vi "Lockin_AIWFM_time.vi"(8 "error in (no error)":errorcluster, 11 "Transport":refnum<class "SMO.Transport.lvclass">) -> (0 "error out":errorcluster, 3 "Transport out":refnum<class "SMO.Transport.lvclass">)   [LabVIEW 2019, in "SMO.Transport.lvclass"]
uses:
  SMO.Transport.lvclass
  <userlib>/LevyLab/Instrument Framework/Instrument Types/Cryostat/Instrument.Cryostat.lvclass
  SMO.Control Experiment/SMO.Control Experiment.lvclass
  <userlib>/LevyLab/Lockin-Multichannel/Instrument.Lockin/Instrument.Lockin.lvclass
  <userlib>/LevyLab/Krohn Hite 7008/Instrument.KH7008.lvclass
  SMO.Control Experiment/Private/Control Experiment SM/Typedefs/Instruments--cluster.ctl
  <userlib>/LevyLab/Instrument Framework/Instrument Types/VSource/Instrument.VSource.lvclass
  <userlib>/LevyLab/Instrument Framework/Instrument Types/VNA/Instrument.VNA.lvclass
  <userlib>/LevyLab/Instrument Framework/Instrument Types/Strain/Instrument.Strain.lvclass
  <userlib>/LevyLab/Instrument Framework/Instrument Types/CBridge/Instrument.CBridge.lvclass
  <vilib>/Waveform/WDTOps.llb/WDT Append Waveforms DBL.vi
  <userlib>/LevyLab/XY Utilities/xy_utilities.lvlib
  <userlib>/LevyLab/XY Utilities/subVIs/Waveform to XY (single).vi
  <userlib>/LevyLab/XY Utilities/subVIs/Get X and Y (single).vi
  <userlib>/LevyLab/Instrument Framework/Instrument Types/Delay Line/Instrument.DelayLine.lvclass
panel:
  in  "Stop":bool
  in  "Tab Control":enum32{"Control", "Waveform", "Other"}(tab)
  in  "wait (ms)":u32=1000
  in  "Experiment Description":string="cool down\n\n"
  in  "Experiment Folder":string="cooldown"
  out "AI":cluster{dbl[], dbl[]}[](graph)
  # "*** These controls are only read if this VI is the top level. If is is called from Sweep Control then the folder and comments come from Sweep Control.vi ***"
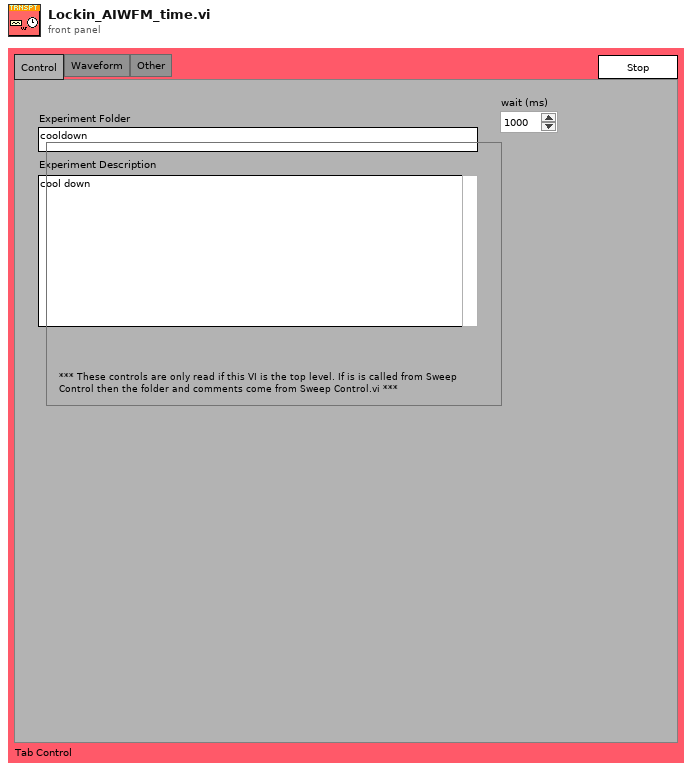
[diagram p1: front panel]
types:
  T1 = enum32{"Invalid", "Standard", "Closed", "Hidden", "Minimized", "Maximized"}
  T2 = enum32{"invalid app kind", "Development System", "Run Time System", "Student Edition", "Embedded LabVIEW", "Evaluation", "Custom"}
  T3 = typedef "SMO.Control Experiment.lvclass/Instruments--cluster.ctl" = cluster{"Lockin":refnum<class "Instrument.Lockin.lvclass">, "Temperature":refnum<class "Instrument.Cryostat.lvclass">, "Magnet":refnum<class "Instrument.Cryostat.lvclass">, "Rotator":refnum<class "Instrument.Cryostat.lvclass">, "Level":refnum<class "Instrument.Cryostat.lvclass">, "C Bridge":refnum<class "Instrument.CBridge.lvclass">, "Optical Delay Line":refnum<class "Instrument.DelayLine.lvclass">, "Strain Cell":refnum<class "Instrument.Strain.lvclass">, "VNA":refnum<class "Instrument.VNA.lvclass">, "Voltage Source":refnum<class "Instrument.VSource.lvclass">, "KH7008":refnum<class "Instrument.KH7008.lvclass">[]}
  T4 = cluster{"Core":cluster{"Current VI Reference":refnum<vi>, "Close Panel on Exit?":bool}, "Transport":refnum<class "SMO.Transport.lvclass">, "Control Experiment":refnum<class "SMO.Control Experiment.lvclass">, "Notifier":refnum<notifier>, "Instruments":T3, "path":path, "time":dbl, "temperature":dbl, "magnet field":dbl, "AI XY (new)":cluster{dbl[], dbl[]}[], "AI XY (all)":cluster{dbl[], dbl[]}[], "AI Waveform (s)":waveform(dbl)[], "t0":timestamp, "Execution:State":enum32{"Bad", "Idle", "Run top level", "Running"}}
  T5 = enum32{"Bad", "Idle", "Run top level", "Running"}
  T6 = cluster{"Current VI Reference":refnum<vi>, "Close Panel on Exit?":bool}
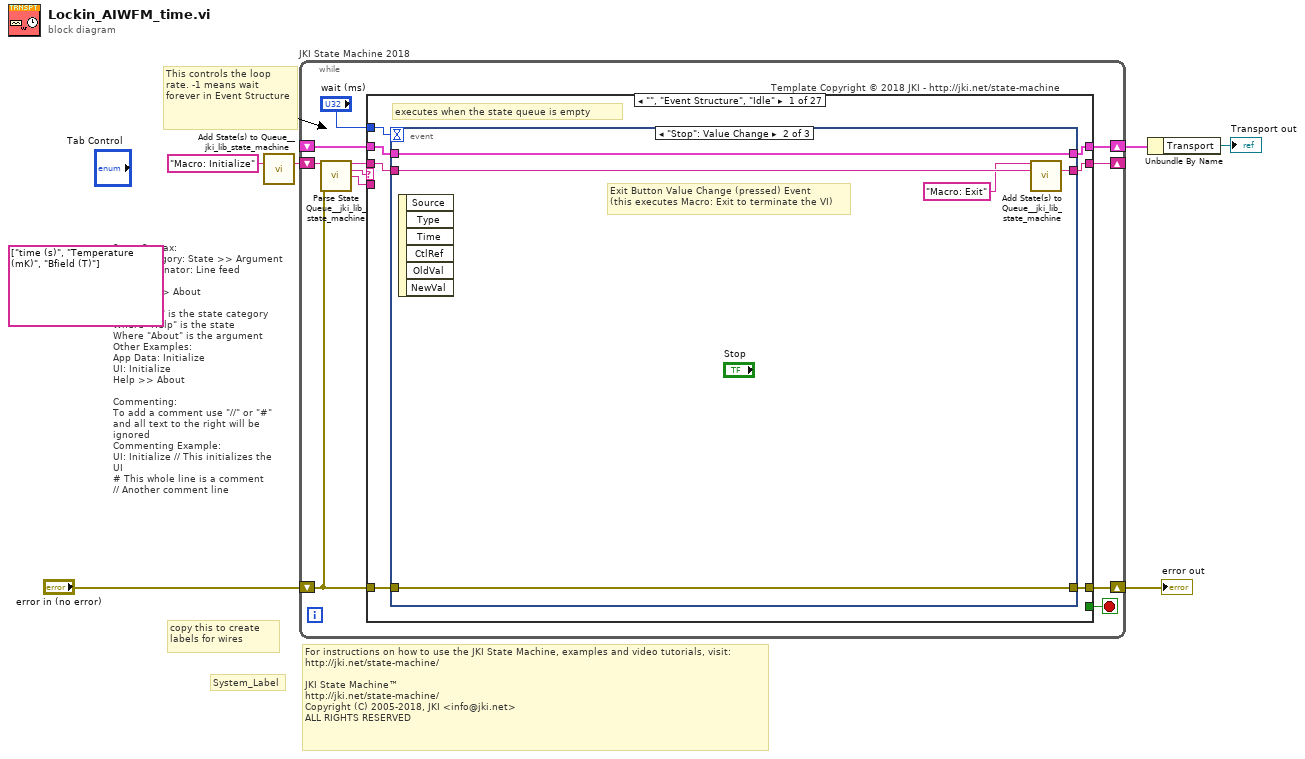
[diagram p0: block diagram]
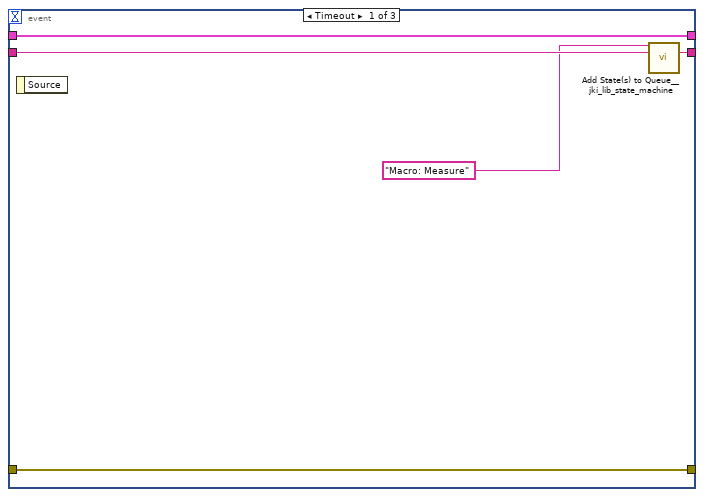
[diagram p2: hidden frame]
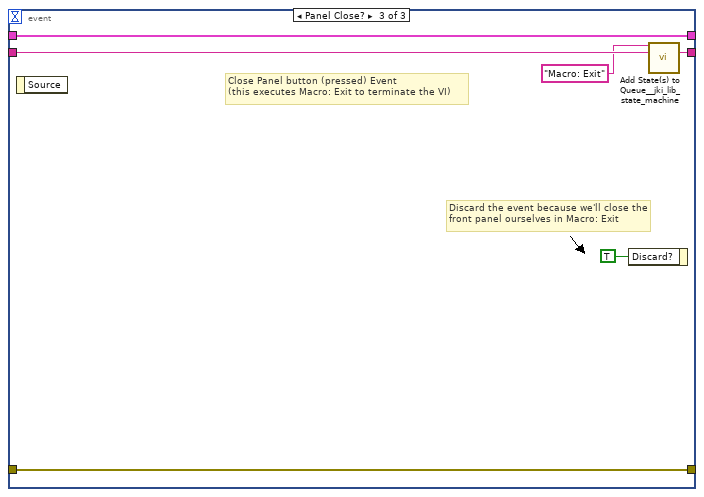
[diagram p3: hidden frame]
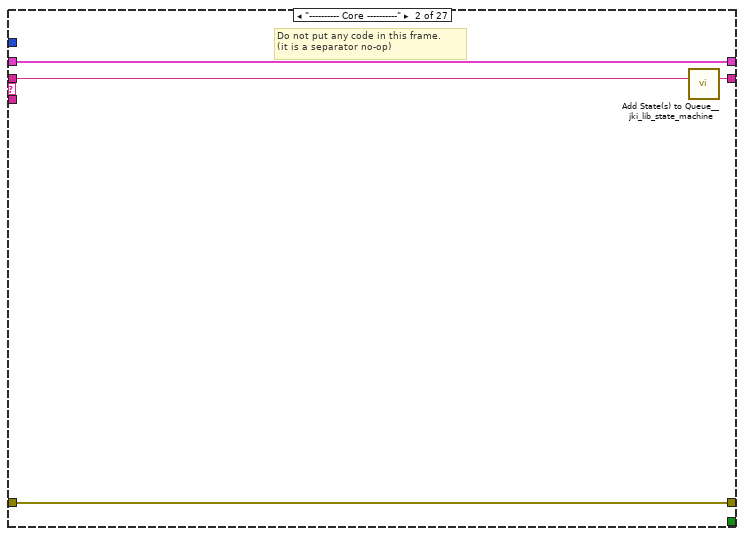
[diagram p4: hidden frame]
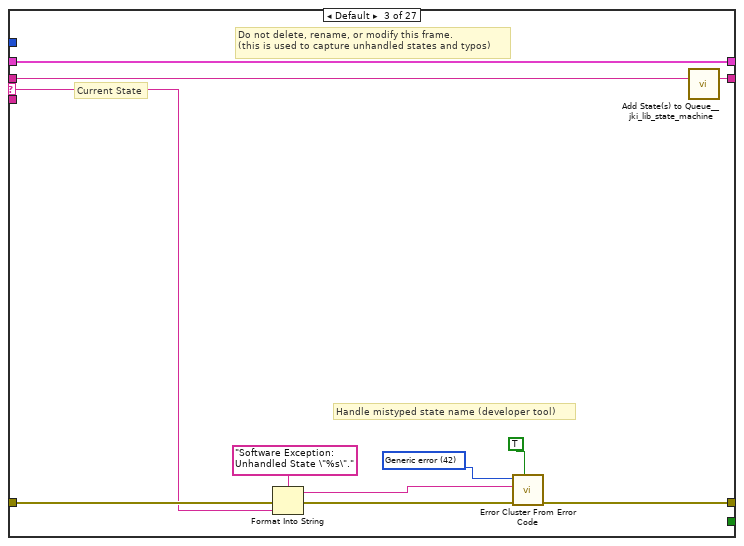
[diagram p5: hidden frame]
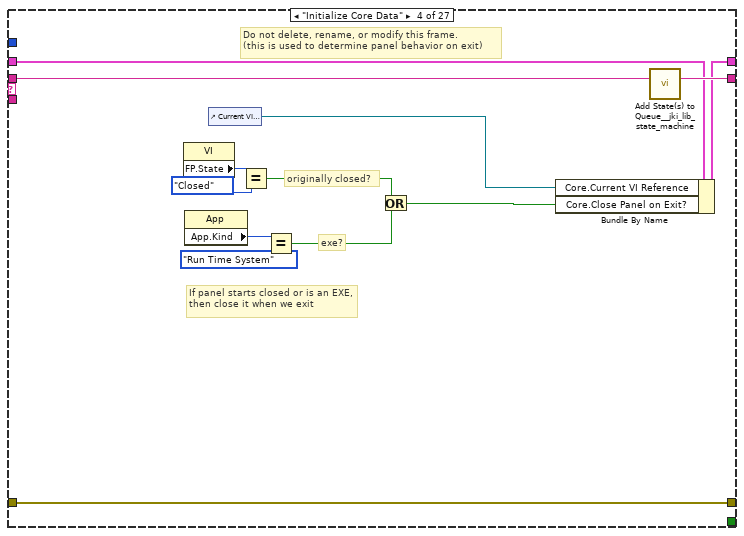
[diagram p6: hidden frame]
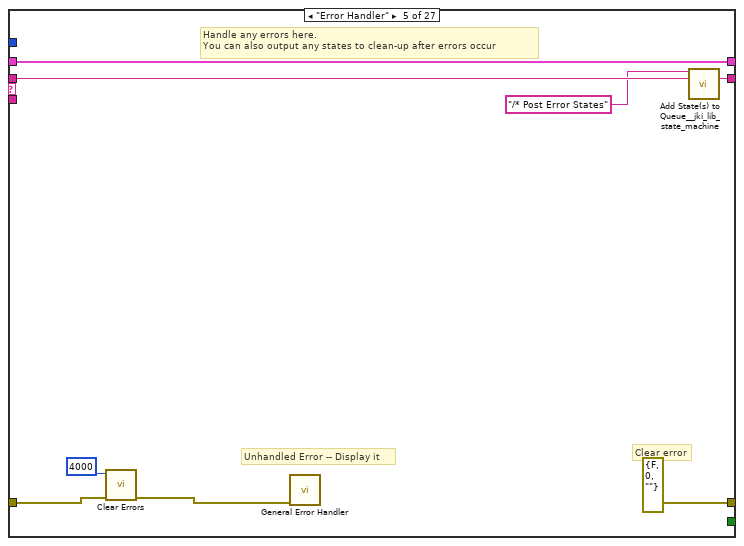
[diagram p7: hidden frame]
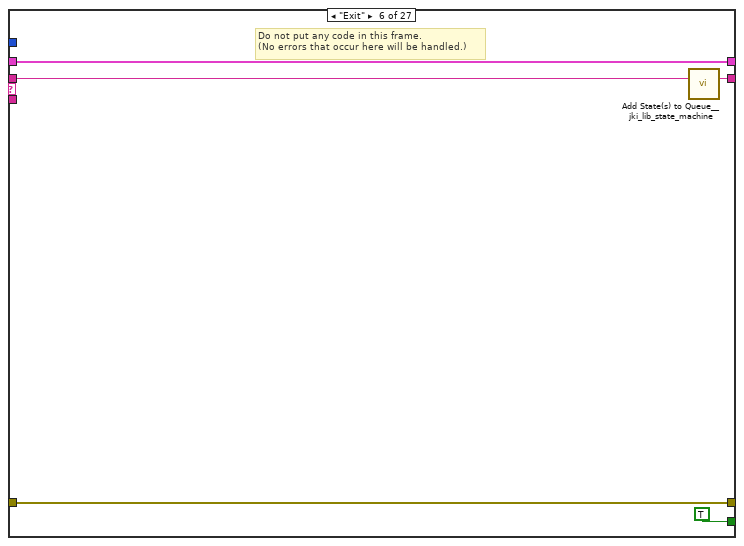
[diagram p8: hidden frame]
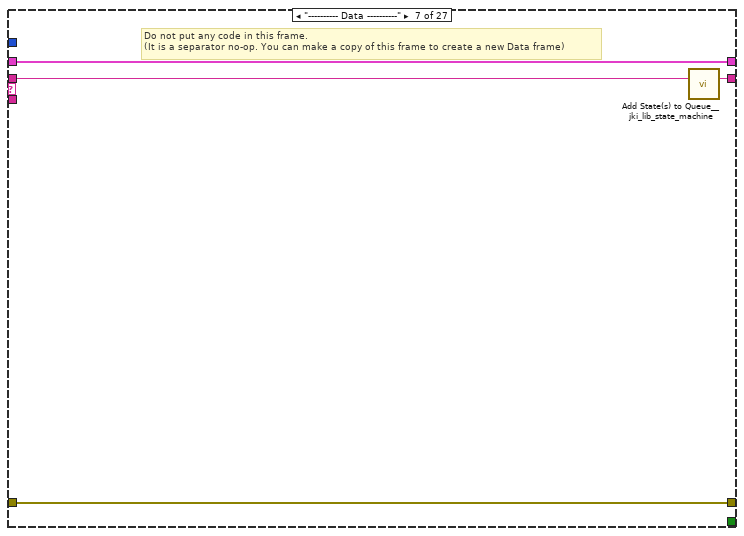
[diagram p9: hidden frame]
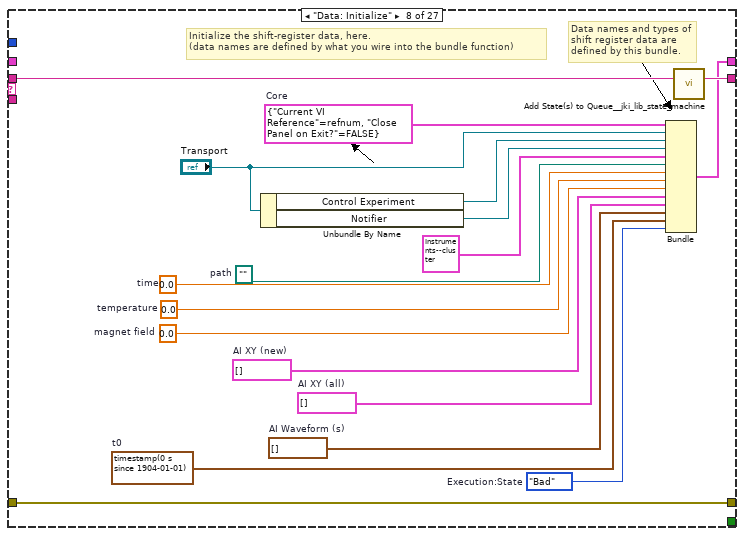
[diagram p10: hidden frame]
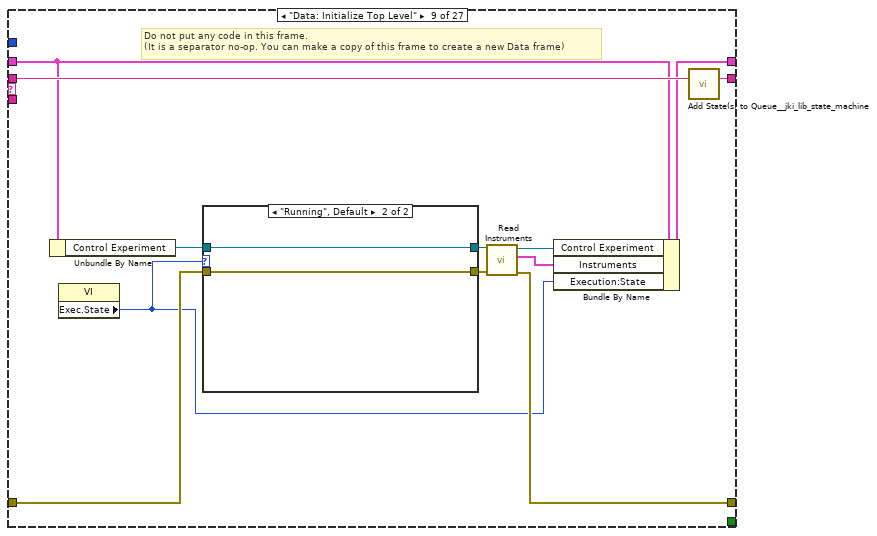
[diagram p11: hidden frame]
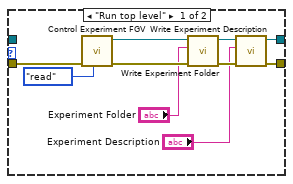
[diagram p12: hidden frame]
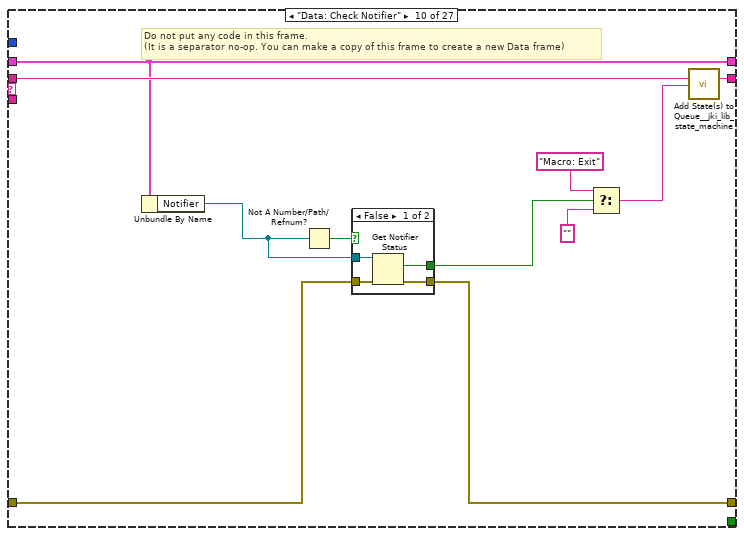
[diagram p13: hidden frame]
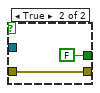
[diagram p14: hidden frame]
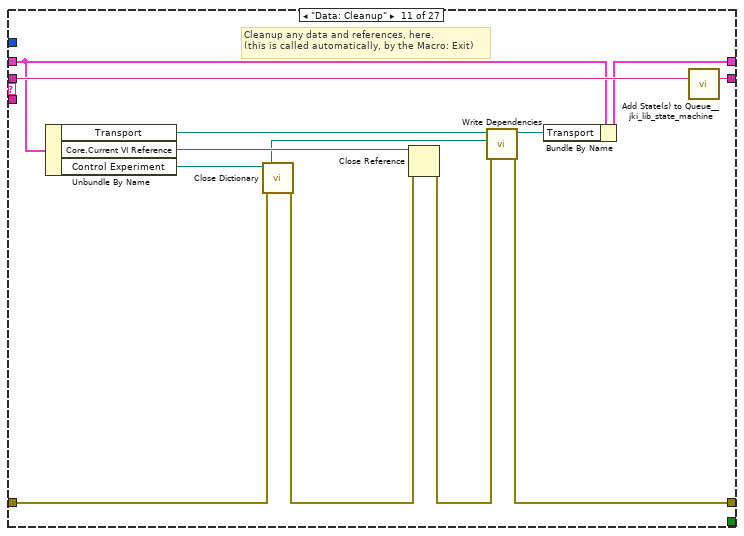
[diagram p15: hidden frame]
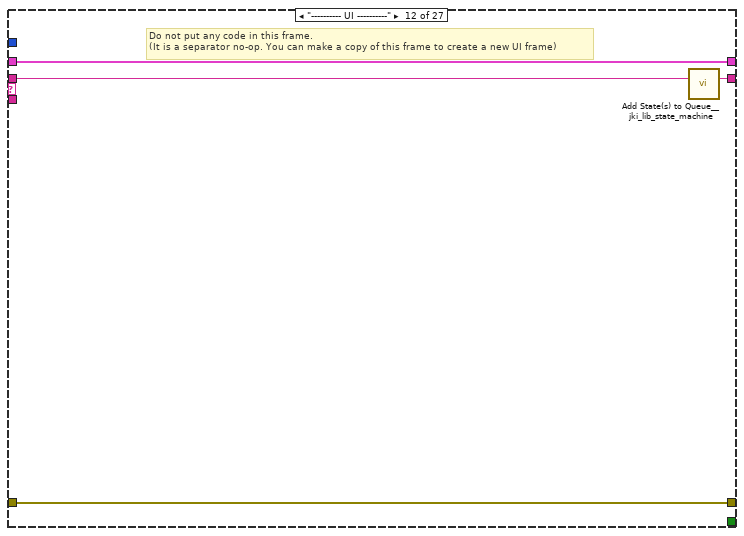
[diagram p16: hidden frame]
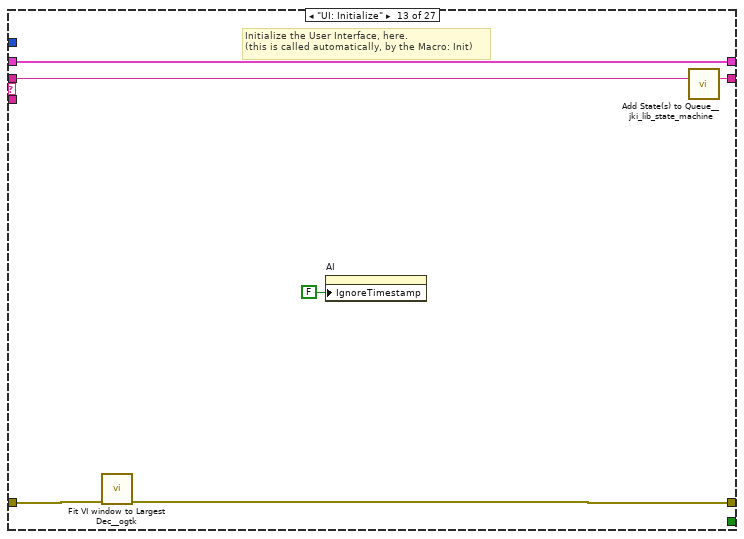
[diagram p17: hidden frame]
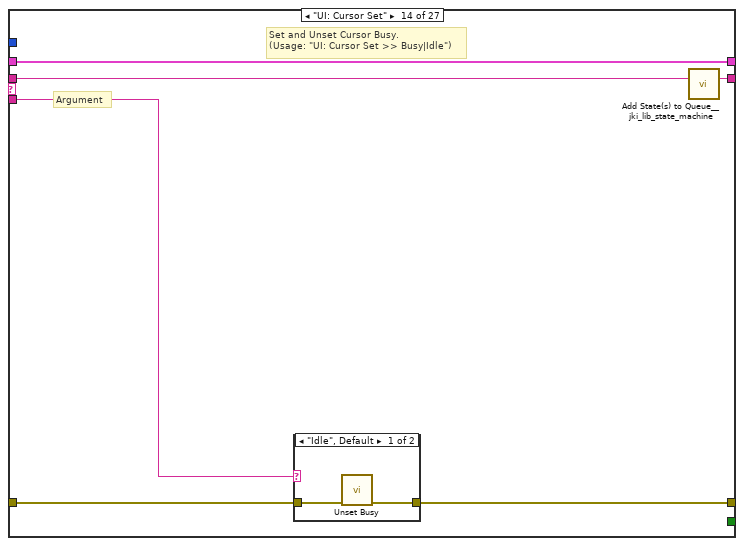
[diagram p18: hidden frame]
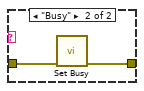
[diagram p19: hidden frame]
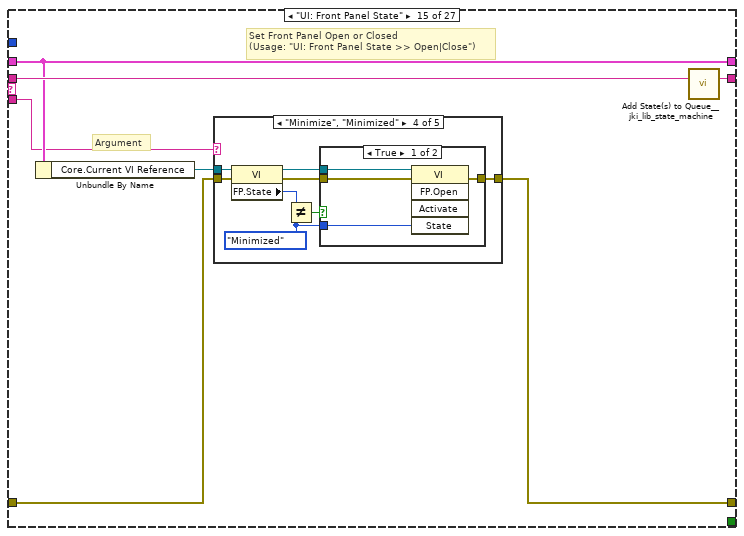
[diagram p20: hidden frame]
diagram:
  (unwired) string[] ["time (s)", "Temperature (mK)", "Bfield (T)"] ("wavenames (.Vx, etc)")
  # "For instructions on how to use the JKI State Machine, examples and video tutorials, visit:\nhttp://jki.net/state-machine/\n\nJKI State Machine™\nhttp://jki.net/state-machine/\nCopyright (C) 2005-2018, JKI <info@jki.net>\nALL RIGHTS RESERVED"
  # "State Syntax:\nStateCategory: State >> Argument\nLine Terminator: Line feed\nExample:\nUI: Help >> About\n\nWhere \"UI\" is the state category\nWhere \"Help\" is the state\nWhere \"About\" is the argument\nOther Examples:\nApp Data: Initialize\nUI: Initialize\nHelp >> About\n\nCommenting:\nTo add a comment use \"//\" or \"#\" and all text to the right will be ignored\nCommenting Example:\nUI: Initialize // This initializes the UI\n# This whole line is a comment\n// Another comment line"
  # "copy this to create labels for wires"
  # "This controls the loop rate. -1 means wait forever in Event Structure"
  # "System_Label"
  n1 = call <vilib>:"Add State(s) to Queue__jki_lib_state_machine.vi"("State(s) in (\"\")"="Macro: Initialize") -> ("States Out"=w6:string)  [unwired: 14 in]
  n2 = while "JKI State Machine 2018" {
    shift-right: [w10] -> w2
    shift-left: _ -> [w9]
    shift-right: [w13] -> w3
    shift-left: "error in (no error)" -> [w8]
    shift-right: [w12] -> _
    shift-left: w6 -> [w14]
    stop <- w11 stop-if-true
    # "Template Copyright © 2018 JKI - http://jki.net/state-machine"
    n3 = call <vilib>:"Parse State Queue__jki_lib_state_machine.vi"("State Queue"=w14, "Error In (no error)"=w8) -> ("Remaining States"=w16:string, "Current State"=w17:string, "Arguments"=w15:string)  [unwired: 11 in]
    n4 = case shown="\"\", \"Event Structure\", \"Idle\"" w17 {
      selector: w17 -> [_ _ w45 _ _ _ _ _ _ _ _ _ _ _ _ _ _ _ _ _ _ _ _ _ _ _ _]
      tunnel: w16 -> [w24 w44 w49 w68 w76 w81 w85 w103 w115 w138 w157 w161 w167 w173 w184 w254 w258 w263 w271 w281 w285 w299 w323 w334 w346 w358 w370]
      tunnel: w15 -> [_ _ _ _ _ _ _ _ _ _ _ _ _ w168 w178 _ _ _ _ _ _ _ _ _ _ _ _]
      tunnel: w9 -> [w22 w41 w47 w61 w73 w79 w82 _ w111 w135 w147 w158 w165 w171 w180 w252 w255 w260 w268 w278 w282 w287 w320 w330 w342 w356 w367]
      tunnel: [w21 w42 w51 w65 errorcluster {"status"=FALSE, "code"=0, "source"=""} ("error out") w78 w83 w100 w105 w133 w148 w159 w163 w169 w181 w251 w256 w261 w269 w279 w283 w297 w321 w324 w335 w351 w361] -> w13
      tunnel: w8 -> [w20 w42 w50 w65 w70 w78 w83 w100 w110 w132 w153 w159 w164 w170 w182 w251 w256 w261 w269 w279 w283 w292 w321 w327 w343 w350 w362]
      tunnel: [w23 w43 w48 w67 w75 w80 w84 w102 w114 w137 w156 w160 w166 w172 w183 w253 w257 w262 w270 w280 w284 w298 w322 w333 w345 w357 w369] -> w12
      tunnel: [_ _ _ _ _ TRUE _ _ _ _ _ _ _ _ _ _ _ _ _ _ _ _ _ _ _ _ _] -> w11
      tunnel: [w19 w41 w47 w66 w73 w79 w82 w101 w112 w135 w146 w158 w165 w171 w180 w252 w255 w260 w268 w278 w282 w286 w320 w331 w341 w355 w368] -> w10
      tunnel: "wait (ms)" -> [w18 _ _ _ _ _ _ _ _ _ _ _ _ _ _ _ _ _ _ _ _ _ _ _ _ _ _]
      frame "", "Event Structure", "Idle" {
        # "executes when the state queue is empty"
        n5 = event shown="[1] \"Stop\": Value Change" {
          selector: _ -> [_ _ _]
          dyn-events: _ -> [_ _ _]
          timeout: w18 -> [_ _ _]
          tunnel: w24 -> [w29 w34 w40]
          tunnel: [w28 w33 w39] -> w23
          tunnel: w22 -> [w26 w31 w37]
          tunnel: [w27 w32 w38] -> w21
          tunnel: w20 -> [w27 w32 w38]
          tunnel: [w26 w31 w37] -> w19
          event Timeout {
            n6 = event-data() -> ()  [unwired: 1 in, 1 out]
            n7 = call <vilib>:"Add State(s) to Queue__jki_lib_state_machine.vi"("State(s) in Front (\"\")"="Macro: Measure" ("State(s) in Front (\"\")"), "State(s) in (\"\")"=w29) -> ("States Out"=w28:string)  [unwired: 13 in]
          }
          event "Stop": Value Change {
            # "Exit Button Value Change (pressed) Event\n(this executes Macro: Exit to terminate the VI)"
            n8 = event-data() -> ()  [unwired: 1 in, 6 out]
            n9 = call <vilib>:"Add State(s) to Queue__jki_lib_state_machine.vi"("State(s) in Front (\"\")"="Macro: Exit", "State(s) in (\"\")"=w34) -> ("States Out"=w33:string)  [unwired: 13 in]
          }
          event Panel Close? {
            # "Discard the event because we'll close the front panel ourselves in Macro: Exit"
            # "Close Panel button (pressed) Event\n(this executes Macro: Exit to terminate the VI)"
            n10 = event-data() -> ()  [unwired: 1 in, 1 out]
            n11 = event-data("Discard?"=TRUE) -> ()  [unwired: 1 in, 1 out]
            n12 = call <vilib>:"Add State(s) to Queue__jki_lib_state_machine.vi"("State(s) in Front (\"\")"="Macro: Exit", "State(s) in (\"\")"=w40) -> ("States Out"=w39:string)  [unwired: 13 in]
          }
        }
      }
      frame "---------- Core ----------" {
        # "Do not put any code in this frame.\n(it is a separator no-op)"
        n13 = call <vilib>:"Add State(s) to Queue__jki_lib_state_machine.vi"("State(s) in (\"\")"=w44) -> ("States Out"=w43:string)  [unwired: 14 in]
      }
      frame Default {
        w54 = 42 items=["No error", "Argument error", "Memory is full", "Out of zone", "End of file", "File already open", "Generic file I/O error", "File not found", "File permission error", "Disk is full", "Duplicate path", "Too many files open", "System feature not enabled", "Resource file not found", "Cannot add resource", "Resource not found", "Image not found", "Image memory error", "Pen does not exist", "Config type invalid", "Config token not found", "Config parse error", "Config memory error", "Bad external code format", "Bad external code offset", "External code not present", "Null window", "Destroy window error", "Null menu", "Print aborted", "Bad print record", "Print driver error", "Windows error during printing", "Memory error during printing", "Print dialog error", "Generic print error", "Invalid device refnum", "Device not found", "Device parameter error", "Device unit error", "Cannot open device", "Device call aborted", "Generic error", "Cancelled by user", "Object ID too low", "Object ID too high", "Object not in heap", "Unknown heap", "Unknown object (invalid DefProc)", "Unknown object (DefProc not in table)", "Message out of range", "Invalid (null) method", "Unknown message", "Manager call not supported", "Bad address", "Network operation in progress", "Network operation timed out", "Connection is busy", "Network attribute not supported", "Network error", "Address in use", "System out of memory", "Connection aborted", "Connection refused", "Not connected", "Already connected", "Connection closed", "Initialization error (interapplication manager)", "Bad occurrence", "Wait on unbound occurrence handler", "Occurrence queue overflow", "Datalog type conflict", "Unused", "Unrecognized type (interapplication manager)", "Memory corrupt", "Failed to make temporary DLL", "Old CIN version", "Drag socket not found", "Failed to load drop-object", "Failed to register OLE object", "Failed to release OLE object", "Format specifier type mismatch", "Unknown format specifier", "Too few format specifiers", "Too many format specifiers", "Scan failed", "Newer CIN version", "Error converting to variant", "Runtime menu error", "Password tampered", "Variant attribute not found", "Incompatible variant data type", "Event data is not available", "Event Store is not present", "Occurrence is not found", "Event Queue is not created", "Event info is not available", "Refnum passed is NULL", "Error retrieving Class GUID", "Error retrieving CoClass GUID", "Error retrieving TypeLib GUID.", "Bad built application magic bytes.", "Specific driver is different from the specific driver associated with the Logical Name.", "There is no session opened to the class driver.", "Max Error", "MAX - Error with config objects", "MAX - Error loading configuration", "MAX - Group not supported"]
        # "Current State"
        # "Do not delete, rename, or modify this frame.\n(this is used to capture unhandled states and typos)"
        # "Handle mistyped state name (developer tool)"
        n14 = Format Into String(format string="Software Exception: Unhandled State \"%s\"." ("message"), error in=w50, w45) -> (resulting string=w53:string, error out=w52:errorcluster)  [unwired: 1 in]
        n15 = call <vilib>:"Error Cluster From Error Code.vi"("show call chain? (False)"=TRUE, "error in (no error)"=w52, "error message (\"\")"=w53, "error code (0)"=w54) -> ("error out"=w51:errorcluster)  [unwired: 5 in]
        n16 = call <vilib>:"Add State(s) to Queue__jki_lib_state_machine.vi"("State(s) in (\"\")"=w49) -> ("States Out"=w48:string)  [unwired: 14 in]
      }
      frame "Initialize Core Data" {
        # "Do not delete, rename, or modify this frame.\n(this is used to determine panel behavior on exit)"
        # "originally closed?"
        # "exe?"
        # "If panel starts closed or is an EXE, then close it when we exit"
        n17 = property class="VI"() -> ("FP.State"=w58:T1)  [unwired: 2 in, 2 out]
        n18 = property class="App"() -> ("App.Kind"=w64:T2)  [unwired: 2 in, 2 out]
        n19 = control-ref of="Current VI Reference"() -> (w59:refnum<vi>)
        n20 = Equal?(x=w58, y=T1."Closed" ("Front Panel Window:State")) -> (x = y?=w56:bool)
        n21 = Equal?(x=w64, y=T2."Run Time System" ("Application:Kind")) -> (x = y?=w62:bool)
        n22 = Or(x=w56, y=w62) -> (x .or. y?=w60:bool)
        n23 = Bundle By Name(cluster=w61, "Core.Current VI Reference"=w59, "Core.Close Panel on Exit?"=w60) -> (w66:T4)
        n24 = call <vilib>:"Add State(s) to Queue__jki_lib_state_machine.vi"("State(s) in (\"\")"=w68) -> ("States Out"=w67:string)  [unwired: 14 in]
      }
      frame "Error Handler" {
        # "Unhandled Error -- Display it"
        # "Handle any errors here.\nYou can also output any states to clean-up after errors occur"
        # "Clear error"
        n25 = call <vilib>:"Clear Errors.vi"("error in (no error)"=w70, "specific error code to clear (0: all)"=4000) -> ("error out"=w69:errorcluster)  [unwired: 4 in, 1 out]
        n26 = call <vilib>:"General Error Handler.vi"("error in (no error)"=w69) -> ()  [unwired: 10 in, 5 out]
        n27 = call <vilib>:"Add State(s) to Queue__jki_lib_state_machine.vi"("State(s) in Front (\"\")"="/* Post Error States", "State(s) in (\"\")"=w76) -> ("States Out"=w75:string)  [unwired: 13 in]
      }
      frame "Exit" {
        # "Do not put any code in this frame.\n(No errors that occur here will be handled.)"
        n28 = call <vilib>:"Add State(s) to Queue__jki_lib_state_machine.vi"("State(s) in (\"\")"=w81) -> ("States Out"=w80:string)  [unwired: 14 in]
      }
      frame "---------- Data ----------" {
        # "Do not put any code in this frame.\n(It is a separator no-op. You can make a copy of this frame to create a new Data frame)"
        n29 = call <vilib>:"Add State(s) to Queue__jki_lib_state_machine.vi"("State(s) in (\"\")"=w85) -> ("States Out"=w84:string)  [unwired: 14 in]
      }
      frame "Data: Initialize" {
        w86 = T5."Bad"  # Execution:State
        w87 = timestamp(0 s since 1904-01-01)  # t0
        w88 = waveform(dbl)[] []  # AI Waveform (s)
        w93 = cluster{dbl[], dbl[]}[] []  # AI XY (new)
        w94 = cluster{dbl[], dbl[]}[] []  # AI XY (all)
        w91 = 0.0  # magnet field
        w90 = 0.0  # temperature
        w89 = 0.0  # time
        w98 = path ""  # path
        w99 = T6 {"Current VI Reference"=refnum, "Close Panel on Exit?"=FALSE}  # Core
        # "Data names and types of shift register data are defined by this bundle."
        # "Initialize the shift-register data, here.\n(data names are defined by what you wire into the bundle function)"
        n30 = Unbundle By Name("Transport") -> ("Control Experiment"=w96:refnum<class "SMO.Control Experiment.lvclass">, "Notifier"=w95:refnum<notifier>)
        n31 = Bundle("Core"=w99, "Transport"="Transport", "Control Experiment"=w96, "Notifier"=w95, "Instruments"=T3 {"Lockin"=refnum, "Temperature"=refnum, "Magnet"=refnum, "Rotator"=refnum, "Level"=refnum, "C Bridge"=refnum, "Optical Delay Line"=refnum, "Strain Cell"=refnum, "VNA"=refnum, "Voltage Source"=refnum, "KH7008"=[]}, "path"=w98, "time"=w89, "temperature"=w90, "magnet field"=w91, "AI XY (new)"=w93, "AI XY (all)"=w94, "AI Waveform (s)"=w88, "t0"=w87, "Execution:State"=w86) -> (w101:T4)  [unwired: 1 in]
        n32 = call <vilib>:"Add State(s) to Queue__jki_lib_state_machine.vi"("State(s) in (\"\")"=w103) -> ("States Out"=w102:string)  [unwired: 14 in]
      }
      frame "Data: Initialize Top Level" {
        # "Do not put any code in this frame.\n(It is a separator no-op. You can make a copy of this frame to create a new Data frame)"
        n33 = Unbundle By Name(w111) -> ("Control Experiment"=w113:refnum<class "SMO.Control Experiment.lvclass">)
        n34 = property class="VI"() -> ("Exec.State"=w104:T5)  [unwired: 2 in, 2 out]
        n35 = case shown="\"Running\", Default" w104 {
          tunnel: w110 -> [w125 w126]
          tunnel: [w120 w126] -> w109
          tunnel: [w119 w127] -> w108
          tunnel: w113 -> [_ w127]
          frame "Run top level" {
            n36 = call "Control Experiment FGV.vi"("Function"=enum16{"read", "write"}."read", "error in (no error)"=w125) -> ("error out"=w123:errorcluster, "Control Experiment out"=w124:refnum<class "SMO.Control Experiment.lvclass">)  [unwired: 8 in]
            n37 = call "Write Experiment Folder.vi"("error in (no error)"=w123, "Experiment Folder"="Experiment Folder", "Control Experiment"=w124) -> ("error out"=w121:errorcluster, "Control Experiment out"=w122:refnum<class "SMO.Control Experiment.lvclass">)  [unwired: 7 in]
            n38 = call "Write Experiment Description.vi"("error in (no error)"=w121, "Experiment Description"="Experiment Description", "Control Experiment"=w122) -> ("error out"=w120:errorcluster, "Control Experiment out"=w119:refnum<class "SMO.Control Experiment.lvclass">)  [unwired: 7 in]
          }
          frame "Running", Default {
          }
        }
        n39 = call "Read Instruments.vi"("error in (no error)"=w109, "Control Experiment"=w108) -> ("error out"=w105:errorcluster, "Instruments"=w106:T3, "Control Experiment out"=w107:refnum<class "SMO.Control Experiment.lvclass">)  [unwired: 7 in]
        n40 = Bundle By Name(cluster=w111, "Control Experiment"=w107, "Instruments"=w106, "Execution:State"=w104) -> (w112:T4)
        n41 = call <vilib>:"Add State(s) to Queue__jki_lib_state_machine.vi"("State(s) in (\"\")"=w115) -> ("States Out"=w114:string)  [unwired: 14 in]
      }
      frame "Data: Check Notifier" {
        # "Do not put any code in this frame.\n(It is a separator no-op. You can make a copy of this frame to create a new Data frame)"
        n42 = Unbundle By Name(w135) -> ("Notifier"=w134:refnum<notifier>)
        n43 = Not A Number/Path/Refnum?(number/path/refnum=w134) -> (NaN/Path/Refnum?=w136:bool)
        n44 = case shown="False" w136 {
          tunnel: [w142 FALSE] -> w131
          tunnel: [w141 w143] -> w133
          tunnel: w134 -> [w140 _]
          tunnel: w132 -> [w139 w143]
          frame False {
            n45 = Get Notifier Status(notifier=w140, error in (no error)=w139) -> (current notification=w142:bool, error out=w141:errorcluster)  [unwired: 3 out]
          }
          frame True {
          }
        }
        n46 = Select(t="Macro: Exit", s=w131, f="") -> (s? t:f=w128:string)
        n47 = call <vilib>:"Add State(s) to Queue__jki_lib_state_machine.vi"("State(s) in (\"\")"=w138, "State(s) at Back (\"\")"=w128) -> ("States Out"=w137:string)  [unwired: 13 in]
      }
      frame "Data: Cleanup" {
        # "Cleanup any data and references, here.\n(this is called automatically, by the Macro: Exit)"
        n48 = Unbundle By Name(w147) -> ("Transport"=w150:refnum<class "SMO.Transport.lvclass">, "Core.Current VI Reference"=w155:refnum<vi>, "Control Experiment"=w154:refnum<class "SMO.Control Experiment.lvclass">)
        n49 = call "Close Dictionary.vi"("error in (no error)"=w153, "Control Experiment"=w154) -> ("error out"=w152:errorcluster, "Control Experiment out"=w145:refnum<class "SMO.Control Experiment.lvclass">)  [unwired: 8 in]
        n50 = Close Reference(reference=w155, error in (no error)=w152) -> (error out=w149:errorcluster)
        n51 = call "Write Dependencies.vi"("error in (no error)"=w149, "Control Experiment"=w145, "Transport in"=w150) -> ("error out"=w148:errorcluster, "Transport out"=w151:refnum<class "SMO.Transport.lvclass">)  [unwired: 7 in]
        n52 = Bundle By Name(cluster=w147, "Transport"=w151) -> (w146:T4)
        n53 = call <vilib>:"Add State(s) to Queue__jki_lib_state_machine.vi"("State(s) in (\"\")"=w157) -> ("States Out"=w156:string)  [unwired: 14 in]
      }
      frame "---------- UI ----------" {
        # "Do not put any code in this frame.\n(It is a separator no-op. You can make a copy of this frame to create a new UI frame)"
        n54 = call <vilib>:"Add State(s) to Queue__jki_lib_state_machine.vi"("State(s) in (\"\")"=w161) -> ("States Out"=w160:string)  [unwired: 14 in]
      }
      frame "UI: Initialize" {
        # "Initialize the User Interface, here.\n(this is called automatically, by the Macro: Init)"
        n55 = call <userlib>:"Fit VI window to Largest Dec__ogtk.vi"("error in (no error)"=w164) -> ("error out"=w163:errorcluster)  [unwired: 5 in, 1 out]
        n56 = property on="AI" class="XYGraph (strict)"("IgnoreTimestamp"=FALSE ("Ignore Timestamp")) -> ()  [unwired: 2 in, 2 out]
        n57 = call <vilib>:"Add State(s) to Queue__jki_lib_state_machine.vi"("State(s) in (\"\")"=w167) -> ("States Out"=w166:string)  [unwired: 14 in]
      }
      frame "UI: Cursor Set" {
        # "Argument"
        # "Set and Unset Cursor Busy.\n(Usage: \"UI: Cursor Set >> Busy|Idle\")"
        n58 = case shown="\"Idle\", Default" w168 {
          tunnel: w170 -> [w175 w177]
          tunnel: [w174 w176] -> w169
          frame "Idle", Default {
            n59 = call <vilib>:"Unset Busy.vi"("error in (no error)"=w175) -> ("error out"=w174:errorcluster)  [unwired: 10 in]
          }
          frame "Busy" {
            n60 = call <vilib>:"Set Busy.vi"("error in (no error)"=w177) -> ("error out"=w176:errorcluster)  [unwired: 9 in, 1 out]
          }
        }
        n61 = call <vilib>:"Add State(s) to Queue__jki_lib_state_machine.vi"("State(s) in (\"\")"=w173) -> ("States Out"=w172:string)  [unwired: 14 in]
      }
      frame "UI: Front Panel State" {
        # "Argument"
        # "Set Front Panel Open or Closed\n(Usage: \"UI: Front Panel State >> Open|Close\")"
        n62 = Unbundle By Name(w180) -> ("Core.Current VI Reference"=w179:refnum<vi>)
        n63 = case shown="\"Minimize\", \"Minimized\"" w178 {
          tunnel: w182 -> [w190 w205 w216 w229 w242]
          tunnel: [w192 w206 w218 w231 w244] -> w181
          tunnel: w179 -> [w191 w203 w217 w230 w243]
          frame "Open", "Standard", Default {
            w185 = T1."Standard" ("State")
            n64 = property class="VI"(reference=w191, error in=w190) -> (reference out=w188:refnum<vi>, error out=w189:errorcluster, "FP.State"=w187:T1)
            n65 = Not Equal?(x=w187, y=w185) -> (x != y?=w186:bool)
            n66 = case shown="True" w186 {
              tunnel: [w196 w198] -> w192
              tunnel: w189 -> [w195 w198]
              tunnel: w188 -> [w194 _]
              tunnel: w185 -> [w193 _]
              frame True {
                n67 = invoke class="VI" method="FP.Open"(reference=w194, error in=w195, "Activate"=TRUE, "State"=w193) -> (error out=w196:errorcluster)  [unwired: 1 in, 4 out]
              }
              frame False {
              }
            }
          }
          frame "Close", "Closed" {
            n68 = property class="VI"(reference=w203, error in=w205) -> (reference out=w202:refnum<vi>, error out=w204:errorcluster, "FP.State"=w200:T1)
            n69 = Not Equal?(x=w200, y=T1."Closed" ("Front Panel Window:State")) -> (x != y?=w199:bool)
            n70 = case shown="True" w199 {
              tunnel: [w207 w210] -> w206
              tunnel: w204 -> [w207 w209]
              tunnel: w202 -> [_ w208]
              frame False {
              }
              frame True {
                n71 = invoke class="VI" method="FP.Close"(reference=w208, error in=w209) -> (error out=w210:errorcluster)  [unwired: 1 in, 2 out]
              }
            }
          }
          frame "Hidden", "Hide" {
            w211 = T1."Hidden" ("State")
            n72 = property class="VI"(reference=w217, error in=w216) -> (reference out=w214:refnum<vi>, error out=w215:errorcluster, "FP.State"=w213:T1)
            n73 = Not Equal?(x=w213, y=w211) -> (x != y?=w212:bool)
            n74 = case shown="True" w212 {
              tunnel: [w222 w223] -> w218
              tunnel: w215 -> [w221 w223]
              tunnel: w214 -> [w220 _]
              tunnel: w211 -> [w219 _]
              frame True {
                n75 = invoke class="VI" method="FP.Open"(reference=w220, error in=w221, "State"=w219) -> (error out=w222:errorcluster)  [unwired: 2 in, 4 out]
              }
              frame False {
              }
            }
          }
          frame "Minimize", "Minimized" {
            w224 = T1."Minimized" ("State")
            n76 = property class="VI"(reference=w230, error in=w229) -> (reference out=w227:refnum<vi>, error out=w228:errorcluster, "FP.State"=w226:T1)
            n77 = Not Equal?(x=w226, y=w224) -> (x != y?=w225:bool)
            n78 = case shown="True" w225 {
              tunnel: [w235 w236] -> w231
              tunnel: w228 -> [w234 w236]
              tunnel: w227 -> [w233 _]
              tunnel: w224 -> [w232 _]
              frame True {
                n79 = invoke class="VI" method="FP.Open"(reference=w233, error in=w234, "State"=w232) -> (error out=w235:errorcluster)  [unwired: 2 in, 4 out]
              }
              frame False {
              }
            }
          }
          frame "Maximize", "Maximized" {
            w237 = T1."Maximized" ("State")
            n80 = property class="VI"(reference=w243, error in=w242) -> (reference out=w240:refnum<vi>, error out=w241:errorcluster, "FP.State"=w239:T1)
            n81 = Not Equal?(x=w239, y=w237) -> (x != y?=w238:bool)
            n82 = case shown="True" w238 {
              tunnel: [w248 w249] -> w244
              tunnel: w241 -> [w247 w249]
              tunnel: w240 -> [w246 _]
              tunnel: w237 -> [w245 _]
              frame True {
                n83 = invoke class="VI" method="FP.Open"(reference=w246, error in=w247, "State"=w245) -> (error out=w248:errorcluster)  [unwired: 2 in, 4 out]
              }
              frame False {
              }
            }
          }
        }
        n84 = call <vilib>:"Add State(s) to Queue__jki_lib_state_machine.vi"("State(s) in (\"\")"=w184) -> ("States Out"=w183:string)  [unwired: 14 in]
      }
      frame "UI: Update Graphs" {
        # "Do not put any code in this frame.\n(It is a separator no-op. You can make a copy of this frame to create a new UI frame)"
        n85 = Unbundle By Name(w252) -> ("AI XY (all)"=→"AI":cluster{dbl[], dbl[]}[])
        n86 = call <vilib>:"Add State(s) to Queue__jki_lib_state_machine.vi"("State(s) in (\"\")"=w254) -> ("States Out"=w253:string)  [unwired: 14 in]
      }
      frame "---------- Macro ----------" {
        # "Do not put any code in this frame.\n(It is a separator no-op. You can make a copy of this frame to create a new Macro frame)"
        n87 = call <vilib>:"Add State(s) to Queue__jki_lib_state_machine.vi"("State(s) in (\"\")"=w258) -> ("States Out"=w257:string)  [unwired: 14 in]
      }
      frame "Macro: Initialize" {
        w259 = "Data: Initialize\nInitialize Core Data\nUI: Initialize\nUI: Front Panel State >> Open\nData: Initialize Top Level"  # Data: Initialize Initialize Core Data UI: Initialize UI: Front Panel State >> Open Data: Initialize Top Level
        # "Initialization Macro\n(This is called once, when the VI starts)"
        n88 = call <vilib>:"Add State(s) to Queue__jki_lib_state_machine.vi"("State(s) in Front (\"\")"=w259, "State(s) in (\"\")"=w263) -> ("States Out"=w262:string)  [unwired: 13 in]
      }
      frame "Macro: Measure" {
        # "Initialization Macro\n(This is called once, when the VI starts)"
        n89 = call <vilib>:"Add State(s) to Queue__jki_lib_state_machine.vi"("State(s) in Front (\"\")"="Measure: Time\nMeasure: Temperature\nMeasure: Magnet\nMeasure: Lockin\nUI: Update Graphs", "State(s) in (\"\")"="File: Save", "State(s) at Back (\"\")"="Data: Check Notifier") -> ("States Out"=w266:string)  [unwired: 12 in]
        n90 = call <vilib>:"Add State(s) to Queue__jki_lib_state_machine.vi"("State(s) in Front (\"\")"=w266, "State(s) in (\"\")"=w271) -> ("States Out"=w270:string)  [unwired: 13 in]
      }
      frame "Macro: Exit" {
        # "Exit Macro\n(This is called once, when the VI exits)"
        n91 = Unbundle By Name(w278) -> ("Core.Close Panel on Exit?"=w277:bool)
        n92 = Select(t="UI: Front Panel State >> Close", s=w277, f="") -> (s? t:f=w274:string)
        n93 = call <vilib>:"Add State(s) to Queue__jki_lib_state_machine.vi"("State(s) in (\"\")"=w274, "State(s) at Back (\"\")"="Data: Cleanup\nExit") -> ("States Out"=w272:string)  [unwired: 13 in]
        n94 = call <vilib>:"Add State(s) to Queue__jki_lib_state_machine.vi"("State(s) in Front (\"\")"=w272, "State(s) in (\"\")"=w281) -> ("States Out"=w280:string)  [unwired: 13 in]
      }
      frame "---------- File ----------" {
        # "Template Separator\n(You can make a copy of, or modify, this frame)"
        n95 = call <vilib>:"Add State(s) to Queue__jki_lib_state_machine.vi"("State(s) in (\"\")"=w285) -> ("States Out"=w284:string)  [unwired: 14 in]
      }
      frame "File: Save" {
        # "Your code here.\n(You can make a copy of, or modify, this frame)"
        n96 = Unbundle By Name(w287) -> ("Execution:State"=w289:T5, "Control Experiment"=w294:refnum<class "SMO.Control Experiment.lvclass">, "AI Waveform (s)"=w295:waveform(dbl)[])
        n97 = for {
          tunnel: w295 -> [w317] mode=indexing
          tunnel: w292 -> [w316]
          shift-right: [w301] -> w293
          shift-left: w294 -> [w312]
          tunnel: [w300] -> w291
          i -> [w309]
          n98 = call-poly <userlib>:"Waveform to XY.vi"("error in (no error)"=w316, "Waveform in"=w317) -> ("error out"=w318:errorcluster, "XY-data out"=w319:cluster{"X-array":dbl[], "Y-array":dbl[]})  [unwired: 8 in]
          n99 = Increment(x=w309) -> (x+1=w311:i32)
          n100 = call-poly <userlib>:"Get X and Y.vi"("error in (no error)"=w318, "XY-data"=w319) -> ("error out"=w303:errorcluster, "Y-array"=w304:dbl[], "X-array"=w305:dbl[])  [unwired: 6 in, 1 out]
          n101 = Format Into String(format string="Ch%d" ("wavenames"), w311) -> (resulting string=w308:string)  [unwired: 2 in, 1 out]
          n102 = Concatenate Strings(w308, "_x" ("string")) -> (w314:string)
          n103 = call "Write Dictionary Element.vi"("error in (no error)"=w303, "value"=w305, "key"=w314, "Control Experiment"=w312) -> ("error out"=w302:errorcluster, "Control Experiment out"=w313:refnum<class "SMO.Control Experiment.lvclass">)  [unwired: 6 in]
          n104 = Concatenate Strings(w308, "_y" ("string")) -> (w315:string)
          n105 = call "Write Dictionary Element.vi"("error in (no error)"=w302, "value"=w304, "key"=w315, "Control Experiment"=w313) -> ("error out"=w300:errorcluster, "Control Experiment out"=w301:refnum<class "SMO.Control Experiment.lvclass">)  [unwired: 6 in]
        }
        n106 = call "Exec State to Append.vi"("Execution:State"=w289) -> ("append?"=w290:bool)  [unwired: 2 in]
        n107 = call "Save Transport TDMS File.vi"("error in (no error)"=w291, "append?"=w290, "Control Experiment"=w293) -> ("error out"=w296:errorcluster, "Control Experiment out"=w288:refnum<class "SMO.Control Experiment.lvclass">)  [unwired: 7 in]
        n108 = Bundle By Name(cluster=w287, "Control Experiment"=w288) -> (w286:T4)
        n109 = call <vilib>:"Clear Errors.vi"("error in (no error)"=w296) -> ("error out"=w297:errorcluster)  [unwired: 5 in, 1 out]
        n110 = call <vilib>:"Add State(s) to Queue__jki_lib_state_machine.vi"("State(s) in (\"\")"=w299) -> ("States Out"=w298:string)  [unwired: 14 in]
      }
      frame "---------- Measure ----------" {
        # "Do not put any code in this frame.\n(It is a separator no-op. You can make a copy of this frame to create a new Macro frame)"
        n111 = call <vilib>:"Add State(s) to Queue__jki_lib_state_machine.vi"("State(s) in (\"\")"=w323) -> ("States Out"=w322:string)  [unwired: 14 in]
      }
      frame "Measure: Time" {
        # "Do not put any code in this frame.\n(It is a separator no-op. You can make a copy of this frame to create a new Macro frame)"
        n112 = Unbundle By Name(w330) -> ("Control Experiment"=w329:refnum<class "SMO.Control Experiment.lvclass">)
        n113 = Get Date/Time In Seconds() -> (seconds since 1Jan1904=w332:timestamp)
        n114 = To Double Precision Float(number=w332) -> (double precision float=w325:dbl)
        n115 = call "Append Dictionary Element.vi"("error in (no error)"=w327, "value"=w325, "key"="Time", "Control Experiment"=w329) -> ("error out"=w324:errorcluster, "Control Experiment out"=w328:refnum<class "SMO.Control Experiment.lvclass">)  [unwired: 6 in]
        n116 = Bundle By Name(cluster=w330, "Control Experiment"=w328) -> (w331:T4)
        n117 = call <vilib>:"Add State(s) to Queue__jki_lib_state_machine.vi"("State(s) in (\"\")"=w334) -> ("States Out"=w333:string)  [unwired: 14 in]
      }
      frame "Measure: Temperature" {
        # "Do not put any code in this frame.\n(It is a separator no-op. You can make a copy of this frame to create a new Macro frame)"
        n118 = Unbundle By Name(w342) -> ("Control Experiment"=w337:refnum<class "SMO.Control Experiment.lvclass">, "Instruments.Temperature"=w344:refnum<class "Instrument.Cryostat.lvclass">)
        n119 = call-dynamic "Get Temperature.vi"("error in (no error)"=w343, "Instrument.Cryostat in"=w344) -> ("error out"=w338:errorcluster, "Temperature (K)"=w339:dbl)  [unwired: 5 in, 3 out]
        n120 = call "Append Dictionary Element.vi"("error in (no error)"=w338, "value"=w339, "key"="Temperature", "Control Experiment"=w337) -> ("error out"=w335:errorcluster, "Control Experiment out"=w336:refnum<class "SMO.Control Experiment.lvclass">)  [unwired: 6 in]
        n121 = Bundle By Name(cluster=w342, "Control Experiment"=w336) -> (w341:T4)
        n122 = call <vilib>:"Add State(s) to Queue__jki_lib_state_machine.vi"("State(s) in (\"\")"=w346) -> ("States Out"=w345:string)  [unwired: 14 in]
      }
      frame "Measure: Magnet" {
        # "Do not put any code in this frame.\n(It is a separator no-op. You can make a copy of this frame to create a new Macro frame)"
        n123 = Unbundle By Name(w356) -> ("Control Experiment"=w353:refnum<class "SMO.Control Experiment.lvclass">, "Instruments.Temperature"=w348:refnum<class "Instrument.Cryostat.lvclass">)
        n124 = call-dynamic "Get Magnet Field.vi"("error in (no error)"=w350, "Instrument.Cryostat in"=w348) -> ("error out"=w349:errorcluster, "B Field (T)"=w347:dbl)  [unwired: 5 in, 3 out]
        n125 = call "Append Dictionary Element.vi"("error in (no error)"=w349, "value"=w347, "key"="Magnet", "Control Experiment"=w353) -> ("error out"=w351:errorcluster, "Control Experiment out"=w352:refnum<class "SMO.Control Experiment.lvclass">)  [unwired: 6 in]
        n126 = Bundle By Name(cluster=w356, "Control Experiment"=w352) -> (w355:T4)
        n127 = call <vilib>:"Add State(s) to Queue__jki_lib_state_machine.vi"("State(s) in (\"\")"=w358) -> ("States Out"=w357:string)  [unwired: 14 in]
      }
      frame "Measure: Lockin" {
        # "Do not put any code in this frame.\n(It is a separator no-op. You can make a copy of this frame to create a new Macro frame)"
        n128 = Unbundle By Name(w367) -> ("t0"=w364:timestamp, "AI Waveform (s)"=w360:waveform(dbl)[], "Instruments.Lockin"=w363:refnum<class "Instrument.Lockin.lvclass">)
        n129 = Array Size(array=w360) -> (size(s)=w359:i32)
        n130 = case shown="Default" w359 {
          tunnel: w360 -> [w374 w393]
          tunnel: [w374 w392] -> w366
          tunnel: [w376 w391] -> w361
          tunnel: w362 -> [w377 w390]
          tunnel: [w372 w386] -> w365
          tunnel: w363 -> [w378 w385]
          tunnel: w364 -> [_ w383]
          frame 0 {
            n131 = for {
              N: 3 -> [_]
              tunnel: w378 -> [w382]
              tunnel: [w379] -> w371
              shift-right: [w380] -> w376
              shift-left: w377 -> [w381]
              n132 = call <userlib>:"waitForNewWaveforms.vi"("error in (no error)"=w381, "Instrument.Lockin in"=w382) -> ("error out"=w380:errorcluster, "Newest AI Waveform"=w379:waveform(dbl)[])  [unwired: 7 in, 1 out]
            }
            n133 = Index Array(array=w371) -> (element=w375:waveform(dbl))  [unwired: 1 in]
            n134 = Unbundle By Name(w375) -> ("t0"=w372:timestamp)
          }
          frame Default {
            n135 = call <userlib>:"getAI.vi"("error in (no error)"=w390, "Instrument.Lockin in"=w385) -> ("error out"=w389:errorcluster, "AI Waveform"=w384:waveform(dbl)[])  [unwired: 7 in, 1 out]
            n136 = Index Array(array=w384) -> (element=w388:waveform(dbl))  [unwired: 1 in]
            n137 = Unbundle By Name(w388) -> ("t0"=w386:timestamp)
            n138 = Equal?(x=w386, y=w383) -> (x = y?=w387:bool)
            n139 = case shown="False" w387 {
              tunnel: w393 -> [w395 w412]
              tunnel: [w398 w412] -> w392
              tunnel: [w397 w413] -> w391
              tunnel: w389 -> [w396 w413]
              tunnel: w384 -> [w399 _]
              frame False {
                n140 = Array Size(array=w395) -> (size(s)=w394:i32)
                n141 = case shown="Default" w394 {
                  tunnel: w399 -> [w401 w406]
                  tunnel: [w401 w405] -> w398
                  tunnel: [w400 w404] -> w397
                  tunnel: w396 -> [w400 w403]
                  tunnel: w395 -> [_ w402]
                  frame 0 {
                  }
                  frame Default {
                    n142 = for {
                      tunnel: w402 -> [w407] mode=indexing
                      tunnel: w406 -> [w411] mode=indexing
                      tunnel: [w410] -> w405 mode=indexing
                      tunnel: [w409] -> w404
                      tunnel: w403 -> [w408]
                      n143 = call-poly <vilib>:"Append Waveforms.vi"("error in (no error)"=w408, "waveform B"=w411, "waveform A"=w407) -> ("error out"=w409:errorcluster, "waveform out"=w410:waveform(dbl))  [unwired: 7 in]
                    }
                  }
                }
              }
              frame True {
              }
            }
          }
        }
        n144 = Bundle By Name(cluster=w367, "t0"=w365, "AI Waveform (s)"=w366) -> (w368:T4)
        n145 = call <vilib>:"Add State(s) to Queue__jki_lib_state_machine.vi"("State(s) in (\"\")"=w370) -> ("States Out"=w369:string)  [unwired: 14 in]
      }
    }
  }
  "error out" <- w3
  n146 = Unbundle By Name(w2) -> ("Transport"=→"Transport out":refnum<class "SMO.Transport.lvclass">)
